vi "Servo_global_test.vi"() -> ()   [LabVIEW 2009, in "Servo.lvlib"]
uses:
  Servo.lvlib
panel:
  out "Array":T1(array[cluster])
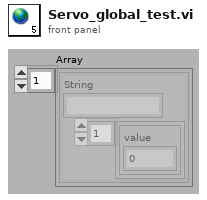
[diagram p1: front panel]
types:
  T1 = cluster{"String":string, cluster{"value":dbl}[]}[]
diagram:
